vi "convert message into string.vi"(7 "add header? (F)":bool, 11 "message":T1 {"id" format="%x"; "data" format="%x"}) -> (0 "status":bool, 1 "error":bool, 2 "message":bool, 3 "message string":string)   [LabVIEW 2024, in "atsj peakcan basic.lvlib"]
uses:
  atsj peakcan basic.lvlib
  message type.ctl
  message.ctl
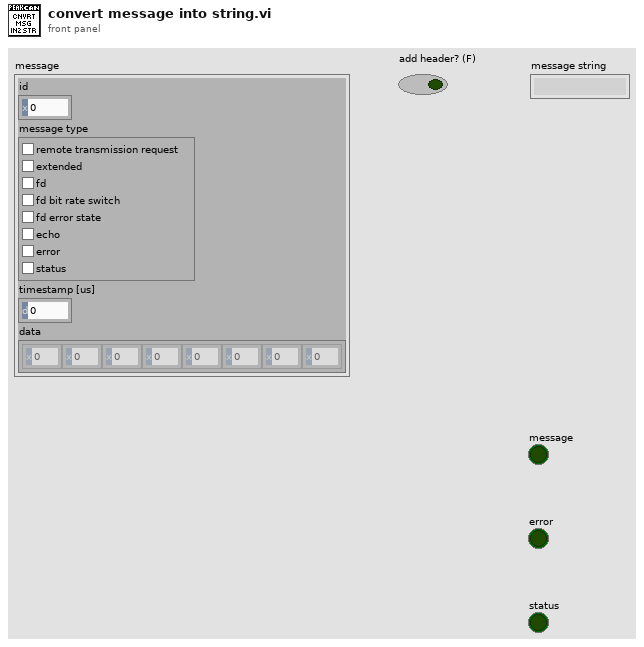
[diagram p1: front panel]
types:
  T1 = typedef "atsj peakcan basic.lvlib/message.ctl" = cluster{"id":u32, "message type":T2, "timestamp [us]":u64, "data":u8[]}
  T2 = typedef "atsj peakcan basic.lvlib/message type.ctl" = cluster{"remote transmission request ":bool, "extended":bool, "fd":bool, "fd bit rate switch":bool, "fd error state":bool, "echo":bool, "error":bool, "status":bool}
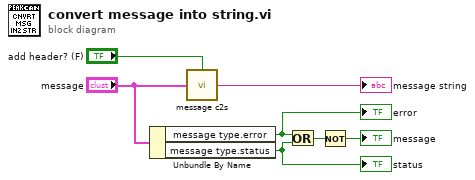
[diagram p0: block diagram]
diagram:
  n1 = Unbundle By Name("message") -> ("message type.error"=w6:bool, "message type.status"=w7:bool)
  "error" <- w6
  "status" <- w7
  n2 = call "message c2s.vi"("cluster"="message", "add header? (F)"="add header? (F)") -> ("string"=→"message string":string)
  n3 = Or(x=w6, y=w7) -> (x .or. y?=w3:bool)
  n4 = Not(x=w3) -> (.not. x?=→"message":bool)
